vi "Get Model Voltages.vi"(8 "error in (no error)":errorcluster, 11 "2230G in":refnum<class "2230G.lvclass">) -> (0 "error out":errorcluster, 3 "2230G out":refnum<class "2230G.lvclass">)   [LabVIEW 2018, in "2230G.lvlib" / "2230G.lvclass"]
uses:
  2230G.lvclass
  2230G.lvclass/2230G.ctl
  PPLs/Power Supply/Parent/Power_Supply.lvlibp/Power Supply.lvclass
  C:/Projects/LabVIEW/PPLs/Power Supply/Parent/Power_Supply.lvlibp/Power Supply.lvclass
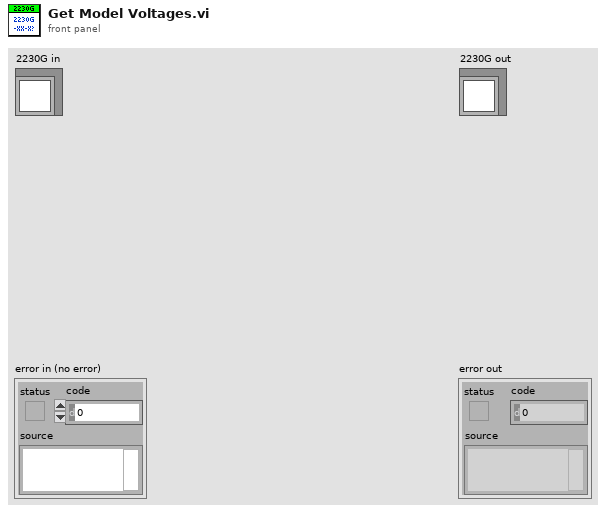
[diagram p1: front panel]
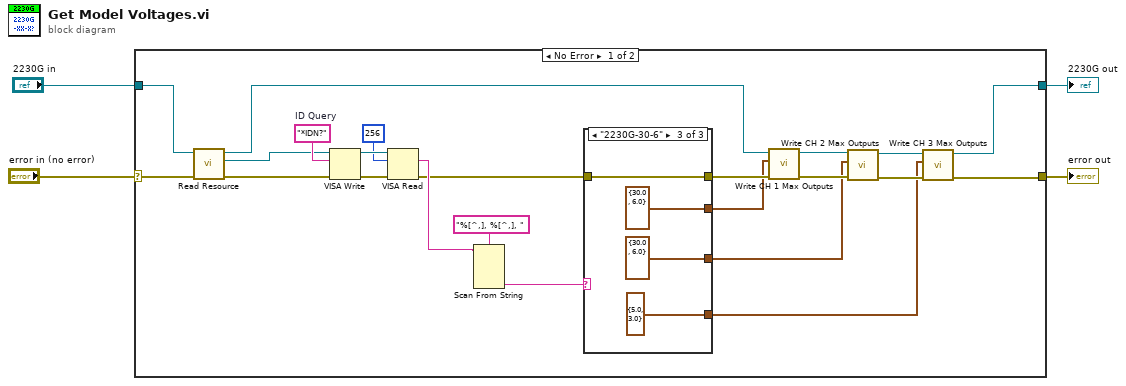
[diagram p0: block diagram]
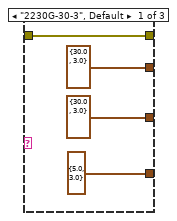
[diagram p2: hidden frame]
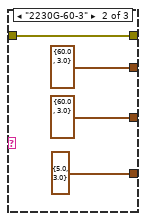
[diagram p3: hidden frame]
diagram:
  n1 = case shown="No Error" "error in (no error)" {
    selector: "error in (no error)" -> [w26 w41]
    tunnel: [w5 w41] -> w3
    tunnel: [w11 w40] -> w1
    tunnel: "2230G in" -> [w27 w40]
    frame No Error {
      w22 = "*IDN?"  # ID Query
      n2 = call "Read Resource.vi"("error in"=w26, "Power Supply in"=w27) -> ("error out"=w19:errorcluster, "Resource"=w20:refnum<visa-resource-name>, "Power Supply out"=w14:refnum<class "2230G.lvclass">)  [unwired: 7 in]
      n3 = VISA Write(VISA resource name=w20, write buffer=w22, error in (no error)=w19) -> (VISA resource name out=w25:refnum<visa-resource-name>, error out=w24:errorcluster)  [unwired: 1 out]
      n4 = VISA Read(VISA resource name=w25, byte count=u32 256, error in (no error)=w24) -> (read buffer=w18:string, error out=w15:errorcluster)  [unwired: 2 out]
      n5 = Scan From String(format string="%[^,], %[^,], ", input string=w18) -> (output 2=w17:string)  [unwired: 2 in, 6 out]
      n6 = case shown="\"2230G-30-6\"" w17 {
        tunnel: [w31 w35 w39] -> w16
        tunnel: w15 -> [w31 w35 w39]
        tunnel: [cluster{"Voltage (V)":dbl, "Current (A)":dbl} {"Voltage (V)"=30.0, "Current (A)"=3.0} ("CH 1 Max Outputs") cluster{"Voltage (V)":dbl, "Current (A)":dbl} {"Voltage (V)"=60.0, "Current (A)"=3.0} ("CH 1 Max Outputs") cluster{"Voltage (V)":dbl, "Current (A)":dbl} {"Voltage (V)"=30.0, "Current (A)"=6.0} ("CH 1 Max Outputs")] -> w8
        tunnel: [cluster{"Voltage (V)":dbl, "Current (A)":dbl} {"Voltage (V)"=30.0, "Current (A)"=3.0} ("CH 2 Max Outputs") cluster{"Voltage (V)":dbl, "Current (A)":dbl} {"Voltage (V)"=60.0, "Current (A)"=3.0} ("CH 2 Max Outputs") cluster{"Voltage (V)":dbl, "Current (A)":dbl} {"Voltage (V)"=30.0, "Current (A)"=6.0} ("CH 2 Max Outputs")] -> w7
        tunnel: [cluster{"Voltage (V)":dbl, "Current (A)":dbl} {"Voltage (V)"=5.0, "Current (A)"=3.0} ("CH 3 Max Outputs") cluster{"Voltage (V)":dbl, "Current (A)":dbl} {"Voltage (V)"=5.0, "Current (A)"=3.0} ("CH 3 Max Outputs") cluster{"Voltage (V)":dbl, "Current (A)":dbl} {"Voltage (V)"=5.0, "Current (A)"=3.0} ("CH 3 Max Outputs")] -> w6
        frame "2230G-30-3", Default {
        }
        frame "2230G-60-3" {
        }
        frame "2230G-30-6" {
        }
      }
      n7 = call "Write CH 1 Max Outputs.vi"("error in (no error)"=w16, "CH 1 Max Outputs"=w8, "2230G in"=w14) -> ("error out"=w10:errorcluster, "2230G out"=w13:refnum<class "2230G.lvclass">)  [unwired: 7 in]
      n8 = call "Write CH 2 Max Outputs.vi"("error in (no error)"=w10, "CH 2 Max Outputs"=w7, "2230G in"=w13) -> ("error out"=w9:errorcluster, "2230G out"=w12:refnum<class "2230G.lvclass">)  [unwired: 7 in]
      n9 = call "Write CH 3 Max Outputs.vi"("error in (no error)"=w9, "CH 3 Max Outputs"=w6, "2230G in"=w12) -> ("error out"=w5:errorcluster, "2230G out"=w11:refnum<class "2230G.lvclass">)  [unwired: 7 in]
    }
    frame Error {
    }
  }
  "error out" <- w3
  "2230G out" <- w1
